vi "Setup Test.vi"(8 "error in (no error)":errorcluster, 11 "CTT Power-Up Test":refnum<class "CTT Power-Up Test.lvclass">) -> (0 "error out":errorcluster, 3 "CTT Power-Up Test":refnum<class "CTT Power-Up Test.lvclass">)   [LabVIEW 2015, in "CTT Power-Up Test.lvclass"]
uses:
  CTT Power-Up Test.lvclass
  Classes/Instruments/Relay Control/Phidget Interface Kit/Class/Phidget Interface Kit 008.lvclass
  Classes/Instruments/MIO Device/MIO Device/Class/typedefs/Channel Type -- Enum.ctl
  Classes/Instruments/MIO Device/MIO Device/Class/MIO Device.lvclass
  Classes/Application/Class/Application.lvclass
  Test Class/Test Class.lvclass
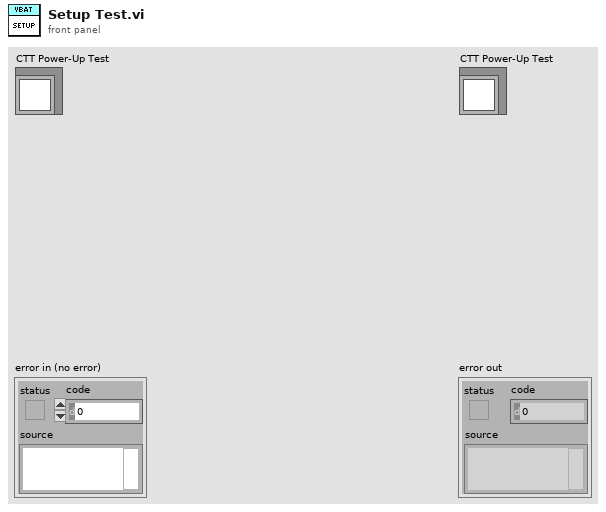
[diagram p1: front panel]
types:
  T1 = typedef "MIO Device.lvlib/MIO Device.lvclass/Channel Type -- Enum.ctl" = enum16{"Analog Input", "Analog Output", "Digital Input", "Digital Output"}
  T2 = cluster{"AI Sample Speed":dbl, "Analog Input Channels":cluster{"Voltage Minimum":dbl, "Voltage Maximum":dbl}[], "Analog Output Channels":cluster{"Voltage Minimum":dbl, "Voltage Maximum":dbl}[], "Digital Channels":cluster{"Output":bool, "Open Collector":bool}[]}
  T3 = typedef "Application.lvlib/App Properties.lvclass/Class Properties -- Cluster.ctl" = cluster{"UUT Info":T4[], "Test Information":refnum<vi>, "Test Complete Event":refnum<user-event>, "Shop Floor System":refnum<class "Shop Floor System.lvclass">, "Gold Board":refnum<class "Golden Board.lvclass">, "Test Recipe":refnum<class "Test Recipe.lvclass">, "Instruments":refnum<class "Instrument.lvclass">[], "Mode":T5, "Test Results":cluster{"Pass":bool[], "Fail Codes":string[]}, "Station Config":refnum<class "Station Config.lvclass">}
  T4 = typedef "Application.lvlib/App Properties.lvclass/UUT Reference -- Cluster.ctl" = cluster{"Serial Number Reference":refnum<vi>, "Status Message Reference":refnum<vi>}
  T5 = typedef "Application.lvlib/Application.lvclass/Op Mode -- Enum.ctl" = u16
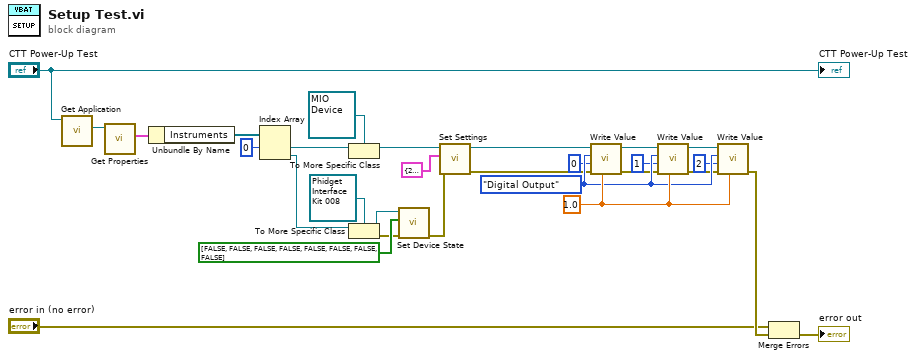
[diagram p0: block diagram]
diagram:
  w25 = Channel_Type_--_Enum."Digital Output" ("Channel Type")
  w26 = 1.0 ("Value (0)")
  n1 = call "Get Application.vi"("Test Class in"="CTT Power-Up Test") -> ("Application.lvlib:Application.lvclass"=w10:refnum<class "Application.lvclass">)  [unwired: 9 in, 1 out]
  n2 = call "Get Properties.vi"("Acrobat Template in"=w10) -> ("Class Properties"=w11:T3)  [unwired: 8 in, 2 out]
  n3 = Unbundle By Name(w11) -> ("Instruments"=w12:refnum<class "Instrument.lvclass">[])
  n4 = Index Array(array=w12, index #1=0 ("index")) -> (element #1=w28:refnum<class "Instrument.lvclass">, element #2=w27:refnum<class "Instrument.lvclass">)  [unwired: 1 in]
  n5 = To More Specific Class(target class=refnum<class "MIO Device.lvclass"> refnum ("MIO Device.lvlib:MIO Device.lvclass"), reference=w28) -> (specific class reference=w9:refnum<class "MIO Device.lvclass">)  [unwired: 1 in, 1 out]
  n6 = To More Specific Class(target class=refnum<class "Phidget Interface Kit 008.lvclass"> refnum ("Phidget Interface Kit 008.lvlib:Phidget Interface Kit 008.lvclass"), reference=w27) -> (specific class reference=w15:refnum<class "Phidget Interface Kit 008.lvclass">, error out=w16:errorcluster)  [unwired: 1 in]
  n7 = call-dynamic "Set Device State.vi"("error in (no error)"=w16, "Device State"=bool[] [FALSE, FALSE, FALSE, FALSE, FALSE, FALSE, FALSE, FALSE] ("Board State"), "Acrobat Template in"=w15) -> ("error out"=w6:errorcluster)  [unwired: 7 in, 1 out]
  n8 = call "Set Settings.vi"("error in (no error)"=w6, "Configuration"=T2 {"AI Sample Speed"=2500.0, "Analog Input Channels"=[{"Voltage Minimum"=-5.0, "Voltage Maximum"=5.0}, {"Voltage Minimum"=-5.0, "Voltage Maximum"=5.0}, {"Voltage Minimum"=-5.0, "Voltage Maximum"=5.0}, {"Voltage Minimum"=-5.0, "Voltage Maximum"=5.0}, {"Voltage Minimum"=-5.0, "Voltage Maximum"=5.0}, {"Voltage Minimum"=-5.0, "Voltage Maximum"=5.0}, {"Voltage Minimum"=-5.0, "Voltage Maximum"=5.0}, {"Voltage Minimum"=-5.0, "Voltage Maximum"=5.0}], "Analog Output Channels"=[{"Voltage Minimum"=-5.0, "Voltage Maximum"=5.0}, {"Voltage Minimum"=-5.0, "Voltage Maximum"=5.0}], "Digital Channels"=[{"Output"=FALSE, "Open Collector"=FALSE}, {"Output"=TRUE, "Open Collector"=FALSE}, {"Output"=FALSE, "Open Collector"=FALSE}, {"Output"=TRUE, "Open Collector"=FALSE}, {"Output"=FALSE, "Open Collector"=FALSE}, {"Output"=TRUE, "Open Collector"=FALSE}, {"Output"=FALSE, "Open Collector"=FALSE}, {"Output"=FALSE, "Open Collector"=FALSE}, {"Output"=FALSE, "Open Collector"=FALSE}, {"Output"=FALSE, "Open Collector"=FALSE}, {"Output"=FALSE, "Open Collector"=FALSE}, {"Output"=FALSE, "Open Collector"=FALSE}, {"Output"=FALSE, "Open Collector"=FALSE}]} ("Default Configuration"), "Acrobat Template in"=w9) -> ("error out"=w5:errorcluster, "Acrobat Template out"=w8:refnum<class "MIO Device.lvclass">)  [unwired: 7 in]
  n9 = call-dynamic "Write Value.vi"("Value (0)"=w26, "error in (no error)"=w5, "Channel (0)"=u32 0, "Channel Type"=w25, "MIO Device in"=w8) -> ("error out"=w23:errorcluster, "MIO Device out"=w22:refnum<class "MIO Device.lvclass">)  [unwired: 5 in]
  n10 = call-dynamic "Write Value.vi"("Value (0)"=w26, "error in (no error)"=w23, "Channel (0)"=u32 1, "Channel Type"=w25, "MIO Device in"=w22) -> ("error out"=w18:errorcluster, "MIO Device out"=w21:refnum<class "MIO Device.lvclass">)  [unwired: 5 in]
  n11 = call-dynamic "Write Value.vi"("Value (0)"=w26, "error in (no error)"=w18, "Channel (0)"=u32 2, "Channel Type"=w25, "MIO Device in"=w21) -> ("error out"=w29:errorcluster)  [unwired: 5 in, 1 out]
  n12 = Merge Errors("error in (no error)", w29) -> (→"error out":errorcluster)
  "CTT Power-Up Test" <- "CTT Power-Up Test"
